vi "oax_GS Order Power Spectrum (Analog Tacho).vi"(0 "scaled signals [EU]":waveform(dbl)[](array[waveform]), 1 "window type":u32, 2 "block size":i32, 3 "dB On":bool, 5 "Waveform":waveform(dbl), 7 "Start":dbl, 9 "Duration":dbl, 11 "error in (no error)":errorcluster, 12 "max order to analyze":dbl, 13 "pulse/rev":i32, 14 "averaging parameters":T2) -> (4 "Order Power Spectrum":T1(array[cluster]), 15 "error out":errorcluster)   [LabVIEW 2017]
uses:
  <vilib>/addons/Sound and Vibration/Order Analysis/Resample Order Tracking/OAT Order Power Spectrum (N Channels).vi
  <vilib>/addons/Sound and Vibration/Order Analysis/Resample Order Tracking/OAT Convert to Even Angle Signal (N Channels).vi
  <vilib>/addons/Sound and Vibration/Order Analysis/Tach Process/OAT Analog Tacho Process (1 Tacho).vi
  <vilib>/Waveform/WDTOps.llb/WDT Get Waveform Subset DBL (LV80).vi
  <vilib>/addons/Sound and Vibration/Order Analysis/Resample Order Tracking/SoundVib_OrderTracking.lvlib
  <vilib>/addons/Sound and Vibration/Order Analysis/Tach Process/SoundVib_TachProcess.lvlib
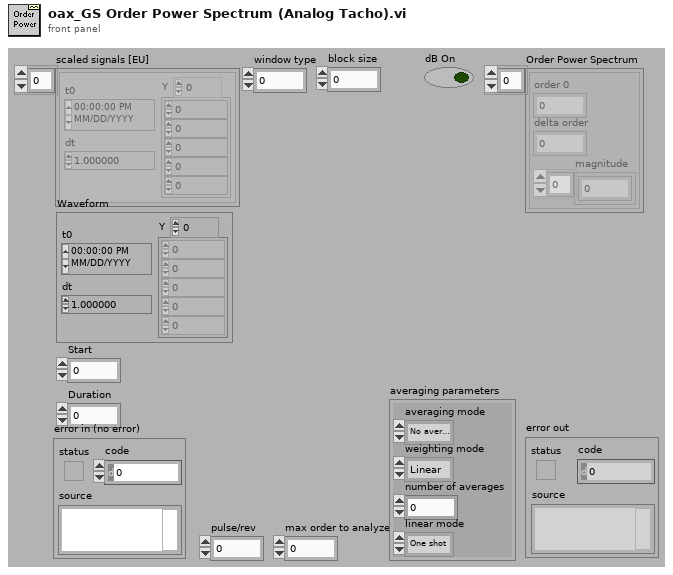
[diagram p1: front panel]
types:
  T1 = cluster{"order 0":dbl, "delta order":dbl, "magnitude":dbl[]}[]
  T2 = cluster{"averaging mode":enum16{"No averaging", "Vector averaging", "RMS averaging", "Peak hold"}, "weighting mode":enum16{"Linear", "Exponential"}, "number of averages":u32, "linear mode":enum16{"One shot", "Auto restart"}}
  T3 = typedef "SoundVib_TachProcess.lvlib/speed profile.ctl" = cluster{"time [s]":dbl[], "speed [RPM]":dbl[]}
  T4 = typedef "svc_Resampled Channel Info.ctl" = cluster{"channel name":string, "description":string, " channel info":T5}
  T5 = typedef "svc_Channel Info.ctl" = cluster{"sensor sensitivity":dbl, "engineering units":T6, "dB reference":dbl, "custom label":string, "weighting filter":T7, "pregain":dbl}
  T6 = typedef "svc_Engineering Units Text Ring.ctl" = u16
  T7 = typedef "svc_Weighting Filter Text Ring.ctl" = u16
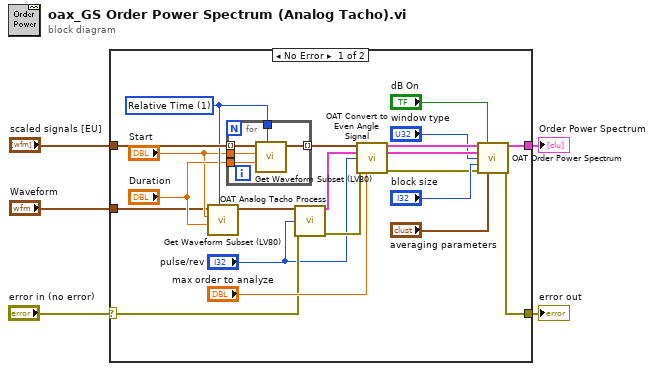
[diagram p0: block diagram]
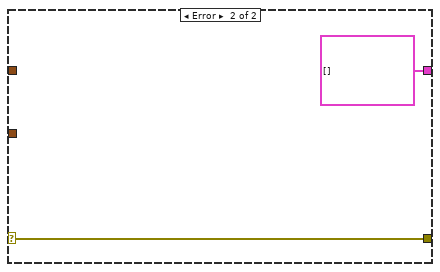
[diagram p2: hidden frame]
diagram:
  n1 = case shown="No Error" "error in (no error)" {
    selector: "error in (no error)" -> [w10 w33]
    tunnel: "scaled signals [EU]" -> [w26 _]
    tunnel: "Waveform" -> [w17 _]
    tunnel: [w11 T1 [] ("order power spectrums")] -> w3
    tunnel: [w7 w33] -> w1
    frame No Error {
      w24 = u16 1 items=["Index", "Relative Time"] ("Mode")
      n2 = call-poly <vilib>:"Get Waveform Subset (LV80).vi"("start/duration format"=w24, "duration"="Duration", "start samples/time"="Start", "waveform in"=w17) -> ("waveform out"=w20:waveform(dbl))  [unwired: 2 in, 3 out]
      n3 = for {
        tunnel: "Start" -> [w31]
        tunnel: "Duration" -> [w30]
        tunnel: w24 -> [w29]
        tunnel: [w28] -> w16 mode=indexing
        tunnel: w26 -> [w27] mode=indexing
        n4 = call-poly <vilib>:"Get Waveform Subset (LV80).vi"("start/duration format"=w29, "duration"=w30, "start samples/time"=w31, "waveform in"=w27) -> ("waveform out"=w28:waveform(dbl))  [unwired: 2 in, 3 out]
      }
      n5 = call-poly <vilib>:"OAT Analog Tacho Process.vi"("analog tacho signal"=w20, "pulse/revolution (1)"="pulse/rev", "error in (no error)"=w10) -> ("speed profile"=w23:T3, "error out"=w9:errorcluster)  [unwired: 8 in, 3 out]
      n6 = call-poly <vilib>:"OAT Convert to Even Angle Signal.vi"("scaled signals [EU]"=w16, "speed profile"=w23, "pulse/revolution (1)"="pulse/rev", "error in (no error)"=w9, "max order (auto)"="max order to analyze") -> ("even-angle signals"=w21:cluster{"r0":dbl, "dr":dbl, "Y":dbl[]}[], "even-angle channel info"=w22:T4[], "error out"=w8:errorcluster)  [unwired: 6 in, 2 out]
      n7 = call-poly <vilib>:"OAT Order Power Spectrum.vi"("even-angle signals"=w21, "dB on? (T)"="dB On", "even-angle channel info"=w22, "window"="window type", "block size"="block size", "error in (no error)"=w8, "averaging parameters"="averaging parameters") -> ("order power spectra"=w11:T1, "error out"=w7:errorcluster)  [unwired: 2 in, 5 out]
    }
    frame Error {
    }
  }
  "Order Power Spectrum" <- w3
  "error out" <- w1
